vi "poistion change.vi"(0 "Value":dbl, 1 "方向":u32, 2 "位置":u32) -> (7 "Data":u8[](array[numeric]))   [LabVIEW 2015]
panel:
  out "Numeric Control":i32
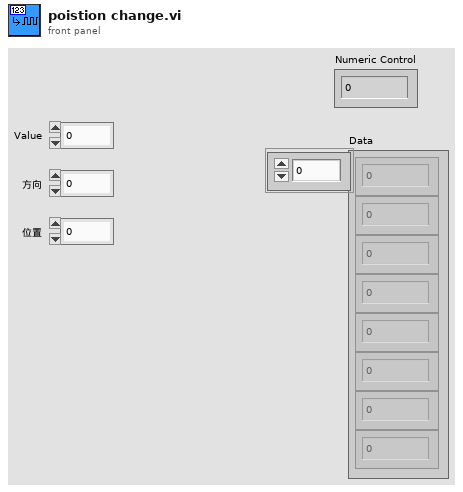
[diagram p1: front panel]
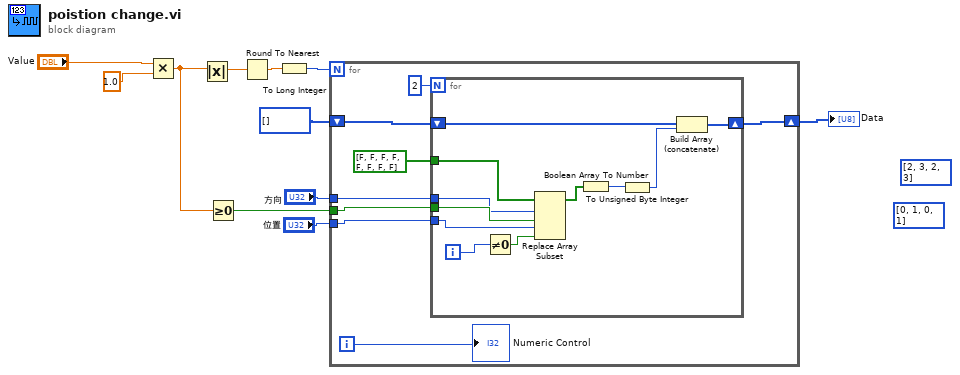
[diagram p0: block diagram]
diagram:
  (unwired) u8[] [0, 1, 0, 1] ("Data")
  (unwired) u8[] [2, 3, 2, 3] ("Data")
  n1 = Multiply(x="Value", y=1.0) -> (x*y=w2:dbl)
  n2 = Absolute Value(x=w2) -> (abs(x)=w11:dbl)
  n3 = Greater Or Equal To 0?(x=w2) -> (x >= 0?=w8:bool)
  n4 = Round To Nearest(number=w11) -> (nearest integer value=w10:dbl)
  n5 = To Long Integer(number=w10) -> (32bit integer=w9:i32)
  n6 = for {
    N: w9 -> [_]
    shift-right: [w17] -> w6
    shift-left: u8[] [] -> [w19]
    tunnel: w8 -> [w18]
    tunnel: "方向" -> [w14]
    tunnel: "位置" -> [w13]
    i -> [w12]
    n7 = for {
      N: 2 -> [_]
      tunnel: w18 -> [w22]
      shift-right: [w26] -> w17
      shift-left: w19 -> [w29]
      tunnel: bool[] [FALSE, FALSE, FALSE, FALSE, FALSE, FALSE, FALSE, FALSE] -> [w23]
      tunnel: w14 -> [w21]
      tunnel: w13 -> [w20]
      i -> [w25]
      n8 = Not Equal To 0?(x=w25) -> (x != 0?=w24:bool)
      n9 = Replace Array Subset(array=w23, new element #1=w22, index #1=w21, new element #2=w24, index #2=w20) -> (w30:bool[])
      n10 = Boolean Array To Number(Boolean array=w30) -> (number=w28:u32)
      n11 = To Unsigned Byte Integer(number=w28) -> (unsigned 8bit integer=w27:u8)
      n12 = Build Array (concatenate)(w29, w27) -> (w26:u8[])
    }
    "Numeric Control" <- w12
  }
  "Data" <- w6
